vi "PathPlanner_ConstraintsZone_Equals.vi"(9 "Other Constraints Zone":T1={"minPosition"=0.0, "maxPosition"=0.0, "Constraints"={"MaxVelocityMps;"=0.0, "MaxAccelerationMpsSq;"=0.0, "MaxAngularVelRadPsEc;"=0.0, "MaxAngularAccRadPSecSq"=0.0, "Exists"=FALSE, "Unlimited"=FALSE, "NominalVoltageVolts"=12.0}, "Present"=FALSE}, 11 "ConstraintsZone":T1={"minPosition"=0.0, "maxPosition"=0.0, "Constraints"={"MaxVelocityMps;"=0.0, "MaxAccelerationMpsSq;"=0.0, "MaxAngularVelRadPsEc;"=0.0, "MaxAngularAccRadPSecSq"=0.0, "Exists"=FALSE, "Unlimited"=FALSE, "NominalVoltageVolts"=12.0}, "Present"=FALSE}) -> (3 "Equal":bool)   [LabVIEW 2019, in "PathPlanner24.lvlib"]
doc: "Compares two Constraints Zone definitions\n\n Inputs:\n -- ConstraintsZone - cluster - first definition to compare\n -- Other ConstraintsZone - cluster - other definition to compare\n\nOutputs:\n -- Equal - boolean - TRUE if equal."
uses:
  PathPlanner24.lvlib
  TypeDef/PathPlannerPathConstraints.ctl
  TypeDef/PathPlannerConstraintsZone.ctl
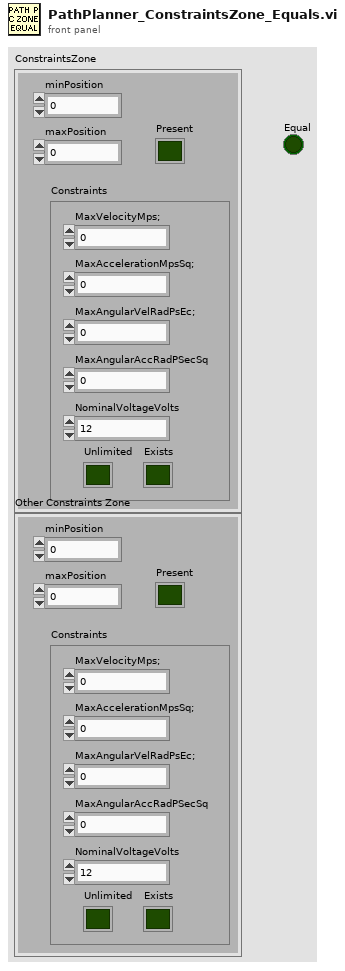
[diagram p1: front panel]
types:
  T1 = typedef "PathPlanner24.lvlib/PathPlannerConstraintsZone.ctl" = cluster{"minPosition":dbl, "maxPosition":dbl, "Constraints":T2, "Present":bool}
  T2 = typedef "PathPlanner24.lvlib/PathPlannerPathConstraints.ctl" = cluster{"MaxVelocityMps;":dbl, "MaxAccelerationMpsSq;":dbl, "MaxAngularVelRadPsEc;":dbl, "MaxAngularAccRadPSecSq":dbl, "Exists":bool, "Unlimited":bool, "NominalVoltageVolts":dbl}
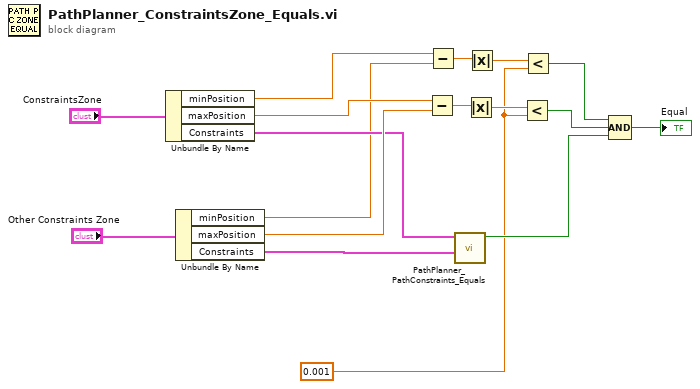
[diagram p0: block diagram]
diagram:
  w2 = 0.001 ("y")
  n1 = Unbundle By Name("ConstraintsZone") -> ("minPosition"=w4:dbl, "maxPosition"=w15:dbl, "Constraints"=w9:T2)
  n2 = Unbundle By Name("Other Constraints Zone") -> ("minPosition"=w3:dbl, "maxPosition"=w14:dbl, "Constraints"=w8:T2)
  n3 = Subtract(x=w15, y=w14) -> (x-y=w13:dbl)
  n4 = Subtract(x=w4, y=w3) -> (x-y=w6:dbl)
  n5 = call "PathPlanner_PathConstraints_Equals.vi"("Other PathPlannerConstraints"=w8, "PathPlannerConstraints"=w9) -> ("Equal"=w7:bool)  [unwired: 9 in]
  n6 = Absolute Value(x=w13) -> (abs(x)=w12:dbl)
  n7 = Absolute Value(x=w6) -> (abs(x)=w5:dbl)
  n8 = Less?(x=w12, y=w2) -> (x < y?=w11:bool)
  n9 = Less?(x=w5, y=w2) -> (x < y?=w1:bool)
  n10 = Compound Arithmetic op=AND(w1, w11, w7) -> (→"Equal":bool)
